vi "goto location.vi"(0 "Image Data":T1) -> ()   [LabVIEW 2013]
uses:
  UberCode 1-25-14/typedefs/vision data.ctl
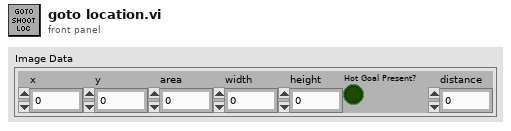
[diagram p1: front panel]
types:
  T1 = typedef "vision data.ctl" = cluster{"x":dbl, "y":dbl, "area":dbl, "width":dbl, "height":dbl, "Hot Goal Present?":bool, "distance":dbl}
  T2 = cluster{"x":bool, "y":bool, "area":bool, "width":bool, "height":bool, "Hot Goal Present?":bool, "distance":bool}
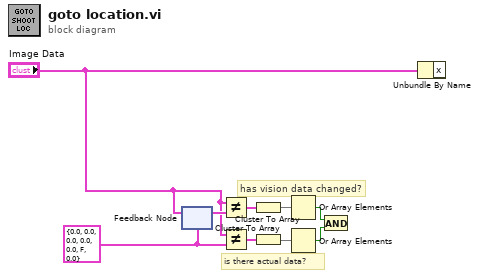
[diagram p0: block diagram]
diagram:
  w1 = T1 {"x"=0.0, "y"=0.0, "area"=0.0, "width"=0.0, "height"=0.0, "Hot Goal Present?"=FALSE, "distance"=0.0} ("Image Data")
  # "is there actual data?"
  # "has vision data changed?"
  n1 = feedback #1(w1) -> (w6:T1)
  n2 = feedback-in #1("Image Data") -> ()
  n3 = Not Equal?(x="Image Data", y=w6) -> (x != y?=w9:T2)
  n4 = Not Equal?(x="Image Data", y=w1) -> (x != y?=w7:T2)
  n5 = Cluster To Array(cluster=w9) -> (array=w8:bool[])
  n6 = Cluster To Array(cluster=w7) -> (array=w4:bool[])
  n7 = Or Array Elements(Boolean array=w8) -> (logical OR=w5:bool)
  n8 = Or Array Elements(Boolean array=w4) -> (logical OR=w3:bool)
  n9 = And(x=w5, y=w3) -> ()  [unwired: 1 out]
  n10 = Unbundle By Name("Image Data") -> ()  [unwired: 1 out]
